vi "零位模式.vi"() -> ()   [LabVIEW 2023]
uses:
  <vilib>/Instr/_visa.llb/VISA Configure Serial Port (Instr).vi
panel:
  in  "+5":bool
  in  "停止":bool
  in  "-5":bool
  out "Write String":string
  out "写入返回数":u32
  out "读取返回数":u32
  out "读取缓冲区":string
  in  "stop bits (10: 1 bit)":u16(ring)=10 caption="停止位（10: 1位）" items=["1.0"=10, "1.5"=15, "2.0"=20]
  in  "parity (0:none)":enum16{"None", "Odd", "Even", "Mark", "Space"}(ring) caption="奇偶（0:无）"
  in  "data bits (8)":u16=8 caption="数据比特(8)" min=5 max=8 step=1
  in  "baud rate (9600)":u32=9600 caption="波特率(9600)"
  in  "VISA resource name":refnum<visa-resource-name> caption="VISA资源名称"
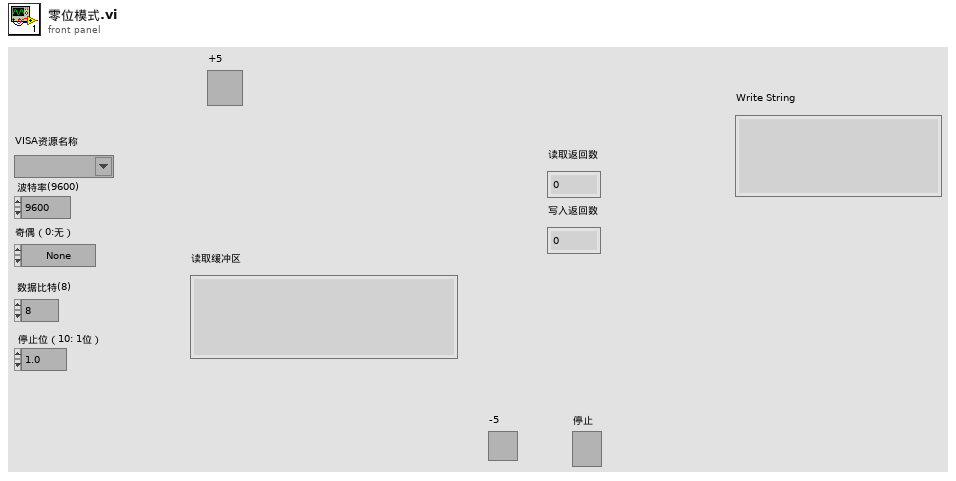
[diagram p1: front panel]
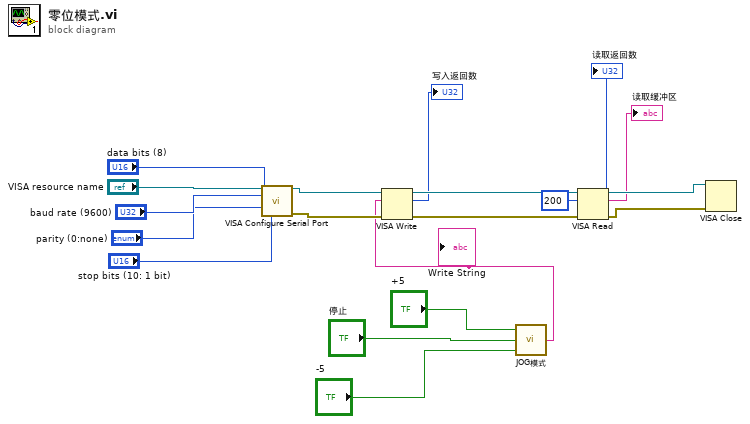
[diagram p0: block diagram]
diagram:
  n1 = call-poly "VISA Configure Serial Port"("VISA resource name"="VISA resource name", "baud rate (9600)"="baud rate (9600)", "data bits (8)"="data bits (8)", "parity (0:none)"="parity (0:none)", "stop bits (10: 1 bit)"="stop bits (10: 1 bit)") -> ("VISA resource name out"=w14:refnum<visa-resource-name>, "error out"=w13:errorcluster)  [unwired: 9 in]
  n2 = call "JOG模式.vi"("-5"="-5", "停止"="停止", "+5"="+5") -> ("Write String"=w4:string)
  "Write String" <- w4
  n3 = VISA Write(VISA resource name=w14, write buffer=w4, error in (no error)=w13) -> (VISA resource name out=w12:refnum<visa-resource-name>, return count=→"写入返回数":u32, error out=w11:errorcluster)
  n4 = VISA Read(VISA resource name=w12, byte count=u32 200 ("字节总数"), error in (no error)=w11) -> (VISA resource name out=w9:refnum<visa-resource-name>, read buffer=→"读取缓冲区":string, return count=→"读取返回数":u32, error out=w8:errorcluster)
  n5 = VISA Close(VISA resource name=w9, error in (no error)=w8) -> ()  [unwired: 1 out]
